vi "JetCU User Interface.vi"() -> ()   [LabVIEW 2017]
uses:
  <vilib>/addons/control/pid/pid.llb/PID (DBL).vi
  <vilib>/addons/control/pid/NI_PID_pid.lvlib
panel:
  out "Process variable and Setpoint":cluster{dbl, "Requested RPM (thousands):":dbl}(graph)
  in  "PID gains":T1={"proportional gain (Kc)"=1.2, "integral time (Ti, min)"=0.1, "derivative time (Td, min)"=0.0} {"derivative time (Td, min)" format="%.3f"; "integral time (Ti, min)" format="%.3f"; "proportional gain (Kc)" format="%.3f"}
  out "Measured RPM (thousands):":dbl(slide)=60.754431603254424 scale=44.0..130.0
  in  "Requested RPM (thousands):":dbl(slide)=60.0 min=0.0 max=0.0 scale=44.0..130.0
  out "Fuel Pump PWM":i32(graph)
  out "Pump Enable":string
  in  "Soft Shut Off":bool
  out "Pump PWM":string
  in  "Send Command":bool
  in  "Custom Command":string
  out "Startup Success":bool
  in  "Output File":path
  in  "Emergency Shut Off":bool
  out "ECU COM Port Out":refnum<visa-resource-name>
  out "Turbine RPM":string
  out "Turbine Temp":string
  out "Error Out":errorcluster
  in  "Error In":errorcluster
  in  "ECU COM Port":refnum<visa-resource-name>
  out "Turbine State":string
  in  "Start Sequence":bool
  # "Note: There are data limits set\non the input to the fuel pump.\nThese were to keep us safe while \ntesting. Look in the PID loop to\nchange anything"
  # "Note: save to a .csv file"
  # "Note: Soft shutoff only works once\nthe startup has completed successfully"
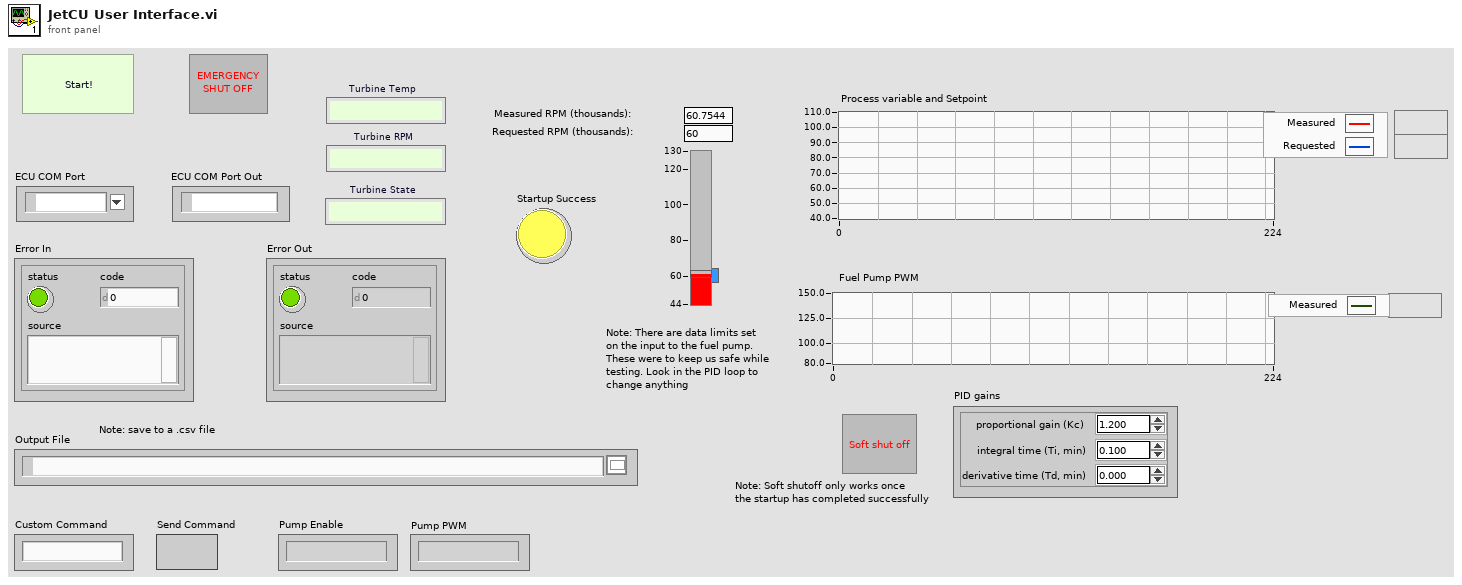
[diagram p1: front panel]
types:
  T1 = cluster{"proportional gain (Kc)":dbl, "integral time (Ti, min)":dbl, "derivative time (Td, min)":dbl}
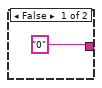
[diagram p3: hidden frame]
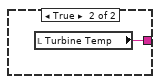
[diagram p4: hidden frame]
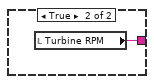
[diagram p5: hidden frame]
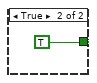
[diagram p8: hidden frame]
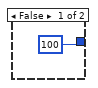
[diagram p9: hidden frame]
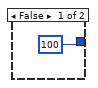
[diagram p10: hidden frame]
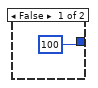
[diagram p11: hidden frame]
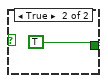
[diagram p12: hidden frame]
diagram:
  w30 = 21 ("Pulse Width")
  w31 = 160 ("Voltage")
  w35 = 16 ("Pulse Width")
  w36 = 160 ("Voltage")
  w27 = 255 ("y")
  w28 = 80 ("y")
  # "Increase fuel\nflow rate"
  # "Waits for the engine to reach\n44000 RPM"
  # "Ramp up the fuel flow rate\naccording to the current RPM.\nWaits until the RPMs reaches 40000"
  # "Ramp up the fuel valve to 66%\nand ramp up the fuel flow rate"
  # "Ramp up the fuel valve to 36%\nand the burner valve to 100%"
  # "Wait for temperature to reach 90 C"
  # "Ramp up the burner valve \nto 59%"
  # "Wait for temperature to reach 25 C"
  # "Update the pump values"
  # "Waits for the turbine to reach 3300 RPM"
  # "If the emergency shutoff button is pressed,\nthe engine will get shut down and the VI\nwill stop"
  # "Reset the Start Sequence\nbutton to false"
  # "Disengage Starter Motor"
  # "Starter Motor 55%"
  # "Start button is inside a while loop that doesn't progess until True"
  # "Fuel Pump Mode 2"
  # "GlowPlugOff"
  # "Start Up\nFuel Pump"
  n1 = call "Initialize Com Port.vi"("Error In"="Error In", "ECU COM Port"="ECU COM Port") -> ("Error Out"=w46:errorcluster, "ECU COM Port Out"=w45:refnum<visa-resource-name>)  [unwired: 8 in]
  n2 = while {
    tunnel: w46 -> [w99]
    tunnel: [w99] -> w44
    stop <- "Start Sequence" stop-if-true
  }
  n3 = call "Initialize Output File.vi"("error in (no error)"=w44, "Output File"="Output File") -> ("error out"=w26:errorcluster)  [unwired: 9 in]
  n4 = flat-sequence {
    tunnel: [w102] -> w25
    tunnel: w26 -> [w102]
    frame #0 {
      w101 = "0" ("Pump Value 1")
      n5 = local write "Pump Enable"(w101) -> ()
      n6 = local write "Pump PWM"(w101) -> ()
    }
  }
  n7 = flat-sequence {
    tunnel: w26 -> [w103]
    tunnel: [w103] -> w40
    frame #0 {
      n8 = local write "Start Sequence"(FALSE ("Strt Sqnc")) -> ()
    }
  }
  n9 = while {
    tunnel: ["Emergency Shut Off"] -> w96
    tunnel: "ECU COM Port" -> [w105]
    stop <- "Emergency Shut Off" stop-if-true
    n10 = case shown="True" "Emergency Shut Off" {
      tunnel: w105 -> [_ w109]
      frame False {
      }
      frame True {
        n11 = call "Emergency Shutoff.vi"("ECU COM Port"=w109) -> ("Error Out"=w108:errorcluster)  [unwired: 9 in, 1 out]
        n12 = local write "Output File"(path "" ("Output File")) -> ()
        n13 = flat-sequence {
          tunnel: w108 -> [w110]
          tunnel: [w110] -> _
          frame #0 {
            n14 = local write "Start Sequence"(FALSE ("Strt Sqnc")) -> ()
          }
        }
      }
    }
  }
  n15 = while {
    tunnel: w25 -> [w129]
    tunnel: w45 -> [w128]
    tunnel: "Output File" -> [w125]
    stop <- w124 continue-if-true
    n16 = call "Get Engine Update.vi"("Error In"=w129, "ECU COM Port"=w128) -> ("Error Out"=w126:errorcluster, "Temperature"=w118:string, "RPMs"=w113:string, "ECU COM Port Out"=w123:refnum<visa-resource-name>)  [unwired: 6 in]
    n17 = call "Time Delay4"() -> ()  [unwired: 11 in, 1 out]
    n18 = call "Safety Check.vi"("Temperature"=w118, "RPMs"=w113) -> ("Safe?"=w124:bool)  [unwired: 9 in]
    n19 = local read "Startup Success"() -> (w112:bool)
    n20 = call "Error Check.vi"("Input"=w113) -> ("Error"=w114:bool)  [unwired: 10 in]
    n21 = call "Error Check.vi"("Input"=w118) -> ("Error"=w117:bool)  [unwired: 10 in]
    n22 = case shown="False" w124 {
      selector: w124 -> [w139 w141]
      tunnel: w123 -> [w140 _]
      tunnel: [w139 w141] -> w122
      frame False {
        n23 = call "Emergency Shutoff.vi"("ECU COM Port"=w140) -> ()  [unwired: 9 in, 2 out]
      }
      frame True {
      }
    }
    n24 = case shown="False" w114 {
      tunnel: w113 -> [w137 _]
      tunnel: [w137 w138] -> w116
      frame False {
        "Turbine RPM" <- w137
      }
      frame True {
        n25 = local read "Turbine RPM"() -> (w138:string)
      }
    }
    n26 = case shown="False" w117 {
      tunnel: w118 -> [w135 _]
      tunnel: [w135 w136] -> w119
      frame False {
        "Turbine Temp" <- w135
      }
      frame True {
        n27 = local read "Turbine Temp"() -> (w136:string)
      }
    }
    n28 = case shown="True" w112 {
      tunnel: ["0" w134] -> w115
      frame False {
      }
      frame True {
        n29 = local read "Requested RPM (thousands):"() -> (w132:dbl)
        n30 = Multiply(x=w132, y=1000.0) -> (x*y=w133:dbl)
        n31 = Number To Decimal String(number=w133) -> (decimal integer string=w134:string)  [unwired: 1 in]
      }
    }
    n32 = Not(x=w122) -> (.not. x?=w127:bool)
    n33 = Stop(stop? (T)=w127) -> ()
    n34 = local read "Pump Enable"() -> (w120:string)
    n35 = local read "Pump PWM"() -> (w121:string)
    n36 = call "Write Data to Output File.vi"("Pump Enable"=w120, "Requested RPM"=w115, "Pump PWM"=w121, "Error In"=w126, "Temperature"=w119, "RPM"=w116, "Output File"=w125) -> ()  [unwired: 4 in, 1 out]
  }
  n37 = call "Set Glow Plug Duty Cycle.vi"("Error In"=w40, "Duty Cycle"=6, "ECU COM Port"=w45) -> ("Error Out"=w88:errorcluster, "ECU COM Port Out"=w85:refnum<visa-resource-name>)  [unwired: 7 in]
  n38 = flat-sequence {
    tunnel: w40 -> [_]
    frame #0 {
      n39 = local write "Turbine State"("Initializing Motor") -> ()
    }
  }
  n40 = while {
    tunnel: w45 -> [w144]
    tunnel: w46 -> [_]
    stop <- FALSE stop-if-true
    n41 = case shown="True" "Send Command" {
      tunnel: "Custom Command" -> [_ w148]
      tunnel: w144 -> [_ w147]
      frame False {
      }
      frame True {
        n42 = call "Time Delay3"() -> ()  [unwired: 11 in, 1 out]
        n43 = VISA Write(VISA resource name=w147, write buffer=w148) -> ()  [unwired: 1 in, 3 out]
      }
    }
  }
  n44 = call "Delay"("error in (no error)"=w88, "Delay Time (s)"=2.0) -> ("error out"=w87:errorcluster)  [unwired: 9 in]
  n45 = call "Set Glow Plug Duty Cycle.vi"("Error In"=w87, "Duty Cycle"=19, "ECU COM Port"=w85) -> ("Error Out"=w86:errorcluster, "ECU COM Port Out"=w81:refnum<visa-resource-name>)  [unwired: 7 in]
  n46 = call "Delay"("error in (no error)"=w86, "Delay Time (s)"=3.0) -> ("error out"=w82:errorcluster)  [unwired: 9 in]
  n47 = call "Set Starter Motor Duty Cycle.vi"("Error In"=w82, "Duty Cycle"=6, "ECU COM Port"=w81) -> ("Error Out"=w80:errorcluster, "ECU COM Port Out"=w78:refnum<visa-resource-name>)  [unwired: 7 in]
  n48 = Stop(stop? (T)=w96) -> ()
  n49 = call "Set Glow Plug Duty Cycle.vi"("Error In"=w80, "Duty Cycle"=15, "ECU COM Port"=w78) -> ("Error Out"=w79:errorcluster, "ECU COM Port Out"=w74:refnum<visa-resource-name>)  [unwired: 7 in]
  n50 = call "Delay"("error in (no error)"=w79, "Delay Time (s)"=3.0) -> ("error out"=w76:errorcluster)  [unwired: 9 in]
  n51 = call "Set Starter Motor Duty Cycle.vi"("Error In"=w76, "Duty Cycle"=4, "ECU COM Port"=w74) -> ("Error Out"=w75:errorcluster, "ECU COM Port Out"=w73:refnum<visa-resource-name>)  [unwired: 7 in]
  n52 = call "Delay"("error in (no error)"=w75, "Delay Time (s)"=0.5) -> ("error out"=w97:errorcluster)  [unwired: 9 in]
  n53 = flat-sequence {
    tunnel: w97 -> [_]
    frame #0 {
      n54 = local write "Turbine State"("Check RPM") -> ()
    }
  }
  n55 = while {
    tunnel: w97 -> [w152]
    tunnel: w73 -> [w151]
    tunnel: [w151] -> w38
    tunnel: [w152] -> w98
    stop <- w155 stop-if-true
    n56 = local read "Turbine RPM"() -> (w150:string)
    n57 = Decimal String To Number(string=w150) -> (number=w154:i32)  [unwired: 2 in, 1 out]
    n58 = Greater Or Equal?(x=w154, y=3300) -> (x >= y?=w156:bool)
    n59 = case shown="False" w156 {
      tunnel: [FALSE TRUE] -> w155
      frame False {
        n60 = call "Delay2"() -> ()  [unwired: 11 in, 1 out]
      }
      frame True {
      }
    }
  }
  n61 = call "Set Pump Fow Rate.vi"("Error In"=w98, "Enable"=w35, "PWM"=w36, "ECU COM Port"=w38) -> ("Error Out"=w39:errorcluster, "ECU COM Port Out"=w37:refnum<visa-resource-name>)  [unwired: 6 in]
  n62 = flat-sequence {
    tunnel: w36 -> [w160]
    tunnel: w35 -> [w159]
    tunnel: w98 -> [_]
    frame #0 {
      n63 = Number To Decimal String(number=w159) -> (decimal integer string=w161:string)  [unwired: 1 in]
      n64 = Number To Decimal String(number=w160) -> (decimal integer string=w162:string)  [unwired: 1 in]
      n65 = local write "Pump Enable"(w161) -> ()
      n66 = local write "Pump PWM"(w162) -> ()
    }
  }
  n67 = call "Set Burner Valve Percent.vi"("Error In"=w39, "Percent"=10, "ECU COM Port"=w37) -> ("Error Out"=w10:errorcluster, "ECU COM Port Out"=w11:refnum<visa-resource-name>)  [unwired: 7 in]
  n68 = while {
    tunnel: [w164] -> w9
    tunnel: w10 -> [w164]
    tunnel: [w163] -> w8
    tunnel: w11 -> [w163]
    stop <- w165 stop-if-true
    n69 = local read "Turbine Temp"() -> (w168:string)
    n70 = Decimal String To Number(string=w168) -> (number=w167:i32)  [unwired: 2 in, 1 out]
    n71 = Greater?(x=w167, y=25) -> (0:w165:bool)
  }
  n72 = for {
    N: 8 -> [_]
    shift-right: [w174] -> _
    shift-left: 27 ("Percent") -> [w176]
    tunnel: w8 -> [w173]
    tunnel: w9 -> [w172]
    tunnel: [w169] -> w17
    tunnel: [w171] -> w18
    n73 = Add(x=w176, y=4 ("Percent")) -> (x+y=w174:i32)
    n74 = call "CmdSeparator"("Delay Time (s)"=0.5) -> ()  [unwired: 10 in, 1 out]
    n75 = call "Set Burner Valve Percent.vi"("Error In"=w172, "Percent"=w174, "ECU COM Port"=w173) -> ("Error Out"=w169:errorcluster, "ECU COM Port Out"=w171:refnum<visa-resource-name>)  [unwired: 7 in]
  }
  n76 = while {
    tunnel: w18 -> [w178]
    tunnel: w17 -> [w179]
    tunnel: [w178] -> w67
    tunnel: [w179] -> w68
    stop <- w182 stop-if-true
    # "Stage2Temp(C)"
    n77 = local read "Turbine Temp"() -> (w177:string)
    n78 = Decimal String To Number(string=w177) -> (number=w180:i32)  [unwired: 2 in, 1 out]
    n79 = Greater Or Equal?(x=w180, y=90) -> (x >= y?=w183:bool)
    n80 = case shown="False" w183 {
      tunnel: [FALSE TRUE] -> w182
      frame False {
        n81 = call "Delay3"() -> ()  [unwired: 11 in, 1 out]
      }
      frame True {
      }
    }
  }
  n82 = flat-sequence {
    tunnel: w17 -> [_]
    frame #0 {
      n83 = local write "Turbine State"("Check Temp") -> ()
    }
  }
  n84 = call "Set Glow Plug Duty Cycle.vi"("Error In"=w68, "Duty Cycle"=0, "ECU COM Port"=w67) -> ("Error Out"=w66:errorcluster, "ECU COM Port Out"=w32:refnum<visa-resource-name>)  [unwired: 7 in]
  n85 = call "CmdSeparator3"("error in (no error)"=w66, "Delay Time (s)"=0.2) -> ("error out"=w29:errorcluster)  [unwired: 9 in]
  n86 = call "Set Pump Fow Rate.vi"("Error In"=w29, "Enable"=w30, "PWM"=w31, "ECU COM Port"=w32) -> ("Error Out"=w34:errorcluster, "ECU COM Port Out"=w33:refnum<visa-resource-name>)  [unwired: 6 in]
  n87 = call "Set Burner Valve Percent.vi"("Error In"=w34, "Percent"=80, "ECU COM Port"=w33) -> ("Error Out"=w63:errorcluster, "ECU COM Port Out"=w64:refnum<visa-resource-name>)  [unwired: 7 in]
  n88 = flat-sequence {
    tunnel: w31 -> [w188]
    tunnel: w30 -> [w187]
    tunnel: w29 -> [_]
    frame #0 {
      n89 = Number To Decimal String(number=w187) -> (decimal integer string=w189:string)  [unwired: 1 in]
      n90 = Number To Decimal String(number=w188) -> (decimal integer string=w190:string)  [unwired: 1 in]
      n91 = local write "Pump Enable"(w189) -> ()
      n92 = local write "Pump PWM"(w190) -> ()
    }
  }
  n93 = call "CmdSeparator18"("error in (no error)"=w63, "Delay Time (s)"=0.75) -> ("error out"=w62:errorcluster)  [unwired: 9 in]
  n94 = call "Set Fuel Valve Percent.vi"("Error In"=w62, "Percent"=12, "ECU COM Port"=w64) -> ("Error Out"=w61:errorcluster, "ECU COM Port Out"=w65:refnum<visa-resource-name>)  [unwired: 7 in]
  n95 = call "CmdSeparator16"("error in (no error)"=w61, "Delay Time (s)"=0.2) -> ("error out"=w94:errorcluster)  [unwired: 9 in]
  n96 = for {
    N: 4 -> [_]
    tunnel: [w192] -> _
    tunnel: [w206] -> _
    tunnel: w65 -> [w198]
    tunnel: w94 -> [w199]
    shift-right: [w197] -> w57
    shift-left: 12 -> [w203]
    shift-right: [w194] -> _
    shift-left: 80 -> [w200]
    tunnel: [w206] -> w55 mode=indexing
    tunnel: [w192] -> w58 mode=indexing
    n97 = Less?(x=w203, y=100) -> (x < y?=w204:bool)
    n98 = Less?(x=w200, y=100) -> (x < y?=w201:bool)
    n99 = case shown="True" w201 {
      tunnel: w200 -> [_ w210]
      tunnel: [100 w208] -> w194
      frame False {
      }
      frame True {
        n100 = Add(x=w210, y=5) -> (x+y=w208:i32)
      }
    }
    n101 = case shown="True" w204 {
      tunnel: w203 -> [_ w214]
      tunnel: [100 w212] -> w197
      frame False {
      }
      frame True {
        n102 = Add(x=w214, y=6) -> (x+y=w212:i32)
      }
    }
    n103 = call "Set Fuel Valve Percent.vi"("Error In"=w199, "Percent"=w197, "ECU COM Port"=w198) -> ("Error Out"=w196:errorcluster, "ECU COM Port Out"=w193:refnum<visa-resource-name>)  [unwired: 7 in]
    n104 = call "Set Burner Valve Percent.vi"("Error In"=w196, "Percent"=w194, "ECU COM Port"=w193) -> ("Error Out"=w195:errorcluster, "ECU COM Port Out"=w192:refnum<visa-resource-name>)  [unwired: 7 in]
    n105 = call "CmdSeparator17"("error in (no error)"=w195, "Delay Time (s)"=0.75) -> ("error out"=w206:errorcluster)  [unwired: 9 in]
  }
  n106 = flat-sequence {
    tunnel: w55 -> [_]
    frame #0 {
      n107 = local write "Turbine State"("Pump Ramp Up") -> ()
    }
  }
  n108 = for {
    N: 3 -> [_]
    tunnel: [w223] -> w48
    tunnel: [w234] -> w49
    shift-right: [w230] -> _
    shift-left: w57 -> [w231]
    tunnel: w55 -> [w227] mode=indexing
    tunnel: w58 -> [w226] mode=indexing
    shift-right: [w219] -> _
    shift-left: 21 -> [w220]
    w218 = 160 ("y")
    n109 = Less?(x=w231, y=100) -> (x < y?=w232:bool)
    n110 = Add(x=w220, y=1) -> (x+y=w219:i32)
    n111 = case shown="True" w232 {
      tunnel: w231 -> [_ w242]
      tunnel: [100 w240] -> w230
      frame False {
      }
      frame True {
        n112 = Add(x=w242, y=10) -> (x+y=w240:i32)
      }
    }
    n113 = call "Set Fuel Valve Percent.vi"("Error In"=w227, "Percent"=w230, "ECU COM Port"=w226) -> ("Error Out"=w229:errorcluster, "ECU COM Port Out"=w228:refnum<visa-resource-name>)  [unwired: 7 in]
    n114 = call "Set Burner Valve Percent.vi"("Error In"=w229, "Percent"=100 ("y"), "ECU COM Port"=w228) -> ("Error Out"=w217:errorcluster, "ECU COM Port Out"=w224:refnum<visa-resource-name>)  [unwired: 7 in]
    n115 = call "Set Pump Fow Rate.vi"("Error In"=w217, "Enable"=w219, "PWM"=w218, "ECU COM Port"=w224) -> ("Error Out"=w222:errorcluster, "ECU COM Port Out"=w223:refnum<visa-resource-name>)  [unwired: 6 in]
    n116 = flat-sequence {
      tunnel: w218 -> [w236]
      tunnel: w219 -> [w235]
      tunnel: w217 -> [_]
      frame #0 {
        n117 = Number To Decimal String(number=w235) -> (decimal integer string=w237:string)  [unwired: 1 in]
        n118 = Number To Decimal String(number=w236) -> (decimal integer string=w238:string)  [unwired: 1 in]
        n119 = local write "Pump Enable"(w237) -> ()
        n120 = local write "Pump PWM"(w238) -> ()
      }
    }
    n121 = call "CmdSeparator20"("error in (no error)"=w222, "Delay Time (s)"=0.5) -> ("error out"=w234:errorcluster)  [unwired: 9 in]
  }
  n122 = call "Set Starter Motor Duty Cycle.vi"("Error In"=w49, "Duty Cycle"=11, "ECU COM Port"=w48) -> ("Error Out"=w14:errorcluster, "ECU COM Port Out"=w15:refnum<visa-resource-name>)  [unwired: 7 in]
  n123 = while {
    tunnel: w15 -> [w248]
    tunnel: w14 -> [w247]
    tunnel: [w246] -> w12
    tunnel: [w245] -> w13
    stop <- w251 stop-if-true
    w250 = 160 ("y")
    n124 = local read "Turbine RPM"() -> (w257:string)
    n125 = Decimal String To Number(string=w257) -> (number=w253:i32)  [unwired: 2 in, 1 out]
    n126 = Multiply(x=w253, y=0.0008) -> (x*y=w255:dbl)
    n127 = call "Set Fuel Valve Percent.vi"("Error In"=w247, "Percent"=100 ("y"), "ECU COM Port"=w248) -> ("Error Out"=w262:errorcluster, "ECU COM Port Out"=w261:refnum<visa-resource-name>)  [unwired: 7 in]
    n128 = Add(x=w255, y=10.537) -> (x+y=w249:dbl)
    n129 = call "Set Burner Valve Percent.vi"("Error In"=w262, "Percent"=0 ("y"), "ECU COM Port"=w261) -> ("Error Out"=w258:errorcluster, "ECU COM Port Out"=w259:refnum<visa-resource-name>)  [unwired: 7 in]
    n130 = call "Set Pump Fow Rate.vi"("Error In"=w258, "Enable"=w249, "PWM"=w250, "ECU COM Port"=w259) -> ("Error Out"=w244:errorcluster, "ECU COM Port Out"=w246:refnum<visa-resource-name>)  [unwired: 6 in]
    n131 = call "CmdSeparator5"("error in (no error)"=w244, "Delay Time (s)"=0.25) -> ("error out"=w245:errorcluster)  [unwired: 9 in]
    n132 = flat-sequence {
      tunnel: w250 -> [w266]
      tunnel: w249 -> [w265]
      tunnel: [w264] -> _
      tunnel: w244 -> [w264]
      frame #0 {
        n133 = Number To Decimal String(number=w265) -> (decimal integer string=w267:string)  [unwired: 1 in]
        n134 = Number To Decimal String(number=w266) -> (decimal integer string=w268:string)  [unwired: 1 in]
        n135 = local write "Pump Enable"(w267) -> ()
        n136 = local write "Pump PWM"(w268) -> ()
      }
    }
    n137 = Greater Or Equal?(x=w253, y=40000) -> (x >= y?=w251:bool)
  }
  n138 = flat-sequence {
    tunnel: w14 -> [_]
    frame #0 {
      n139 = local write "Turbine State"("Ramp Up to Idle") -> ()
    }
  }
  n140 = call "Set Pump Fow Rate.vi"("Error In"=w13, "Enable"=w27, "PWM"=w28, "ECU COM Port"=w12) -> ("Error Out"=w16:errorcluster, "ECU COM Port Out"=w54:refnum<visa-resource-name>)  [unwired: 6 in]
  n141 = flat-sequence {
    tunnel: w28 -> [w272]
    tunnel: w27 -> [w271]
    tunnel: w16 -> [w270]
    tunnel: [w270] -> _
    frame #0 {
      n142 = Number To Decimal String(number=w271) -> (decimal integer string=w273:string)  [unwired: 1 in]
      n143 = Number To Decimal String(number=w272) -> (decimal integer string=w274:string)  [unwired: 1 in]
      n144 = local write "Pump Enable"(w273) -> ()
      n145 = local write "Pump PWM"(w274) -> ()
    }
  }
  n146 = while {
    tunnel: w16 -> [w276]
    tunnel: w54 -> [w275]
    tunnel: [w276] -> w51
    tunnel: [w275] -> w53
    stop <- w277 stop-if-true
    n147 = local read "Turbine RPM"() -> (w280:string)
    n148 = Decimal String To Number(string=w280) -> (number=w279:i32)  [unwired: 2 in, 1 out]
    n149 = Greater?(x=w279, y=44000) -> (0:w277:bool)
  }
  n150 = flat-sequence {
    tunnel: w51 -> [_]
    frame #0 {
      n151 = local write "Turbine State"("Normal Operation") -> ()
    }
  }
  n152 = call "Set Starter Motor Duty Cycle.vi"("Error In"=w51, "Duty Cycle"=0, "ECU COM Port"=w53) -> ("Error Out"=w23:errorcluster, "ECU COM Port Out"=w24:refnum<visa-resource-name>)  [unwired: 7 in]
  n153 = flat-sequence {
    tunnel: w23 -> [_]
    frame #0 {
      "Startup Success" <- TRUE
    }
  }
  n154 = while {
    tunnel: [w298] -> w22
    tunnel: [w297] -> w21
    tunnel: w24 -> [w295]
    tunnel: w23 -> [w296]
    stop <- "Soft Shut Off" stop-if-true
    # "Note: There are data limits on this VI!\nWe added these limits to make sure we\nwere safe during our testing, but they\ncan be deleted to get the engine to run\nfaster"
    # "Control loop using PID"
    n155 = local read "Turbine RPM"() -> (w294:string)
    n156 = Decimal String To Number(string=w294) -> (number=w291:i32)  [unwired: 2 in, 1 out]
    n157 = Divide(x=w291, y=1000) -> (x/y=w283:dbl)
    "Measured RPM (thousands):" <- w283
    n158 = Wait Until Next ms Multiple(millisecond multiple=u32 500 ("unsigned 32bit integer")) -> ()  [unwired: 1 out]
    n159 = call-poly <vilib>:"PID.vi"("output range"=cluster{"output high":dbl, "output low":dbl} {"output high"=20.0, "output low"=-20.0}, "PID gains"="PID gains", "process variable"=w283, "setpoint"="Requested RPM (thousands):") -> ("output"=w287:dbl)  [unwired: 6 in, 1 out]
    n160 = Add(x=w283, y=w287) -> (x+y=w286:dbl)
    n161 = Multiply(x=w286, y=1000.0) -> (x*y=w285:dbl)
    n162 = Bundle(w283, "Requested RPM (thousands):"="Requested RPM (thousands):") -> (→"Process variable and Setpoint":cluster{dbl, "Requested RPM (thousands):":dbl})  [unwired: 1 in]
    n163 = call "RPM to Fuel Flow.vi"("Requested RPM"=w285) -> ("Fuel Pump PWM"=w288:i32)  [unwired: 10 in]
    "Fuel Pump PWM" <- w288
    n164 = Number To Decimal String(number=w288) -> (decimal integer string=→"Pump PWM":string)  [unwired: 1 in]
    n165 = call "Set Pump Fow Rate.vi"("Error In"=w296, "Enable"=255 ("Pulse Width"), "PWM"=w288, "ECU COM Port"=w295) -> ("Error Out"=w297:errorcluster, "ECU COM Port Out"=w298:refnum<visa-resource-name>)  [unwired: 6 in]
    n166 = local write "Pump Enable"("255" ("Pump Value 2")) -> ()
  }
  n167 = call "Emergency Shutoff.vi"("Error In"=w21, "ECU COM Port"=w22) -> ("Error Out"=w42:errorcluster, "ECU COM Port Out"=→"ECU COM Port Out":refnum<visa-resource-name>)  [unwired: 8 in]
  n168 = flat-sequence {
    tunnel: w42 -> [w306]
    tunnel: [w306] -> w95
    frame #0 {
      w305 = "0"
      n169 = local write "Pump Enable"(w305) -> ()
      n170 = local write "Pump PWM"(w305) -> ()
    }
  }
  "Error Out" <- w95
